vi "To 1D Float Tree Data.vi"(10 "1D Flt":dbl[](array[numeric])) -> (3 "1D Flt Tree Data":refnum<class "1D Flt.lvclass">)   [LabVIEW 2017, in "Tree API.lvlib" / "1D Flt.lvclass"]
doc: "Convert a 1D Float value to Tree Data type."
uses:
  1D Flt.lvclass
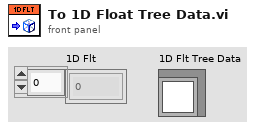
[diagram p1: front panel]
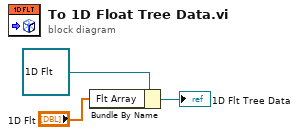
[diagram p0: block diagram]
diagram:
  n1 = Bundle By Name(cluster=refnum<class "1D Flt.lvclass"> refnum ("Flt Array.lvclass"), "Flt Array"="1D Flt") -> (→"1D Flt Tree Data":refnum<class "1D Flt.lvclass">)
